vi "camara.vi"() -> ()   [LabVIEW 2010]
uses:
  <vilib>/addons/PixeLINK/Low Level Functions/ACQUISITION.llb/TDPU-Acquisition-StreamState.ctl
  <vilib>/addons/PixeLINK/Low Level Functions/CAMERA_FEATURES.llb/TDPU-CameraFeatures-FeatureIds.ctl
panel:
  out "output array":u8[][](array[numeric])
  out "unsigned 32bit integer":u32
  out "ROI y":dbl
  out "ROI x":dbl
  in  "Error IN":errorcluster
  out "Error OUT":errorcluster
  in  "error in (no error)":errorcluster
  out "error out":errorcluster
  out "Image":T1(plugin-control)
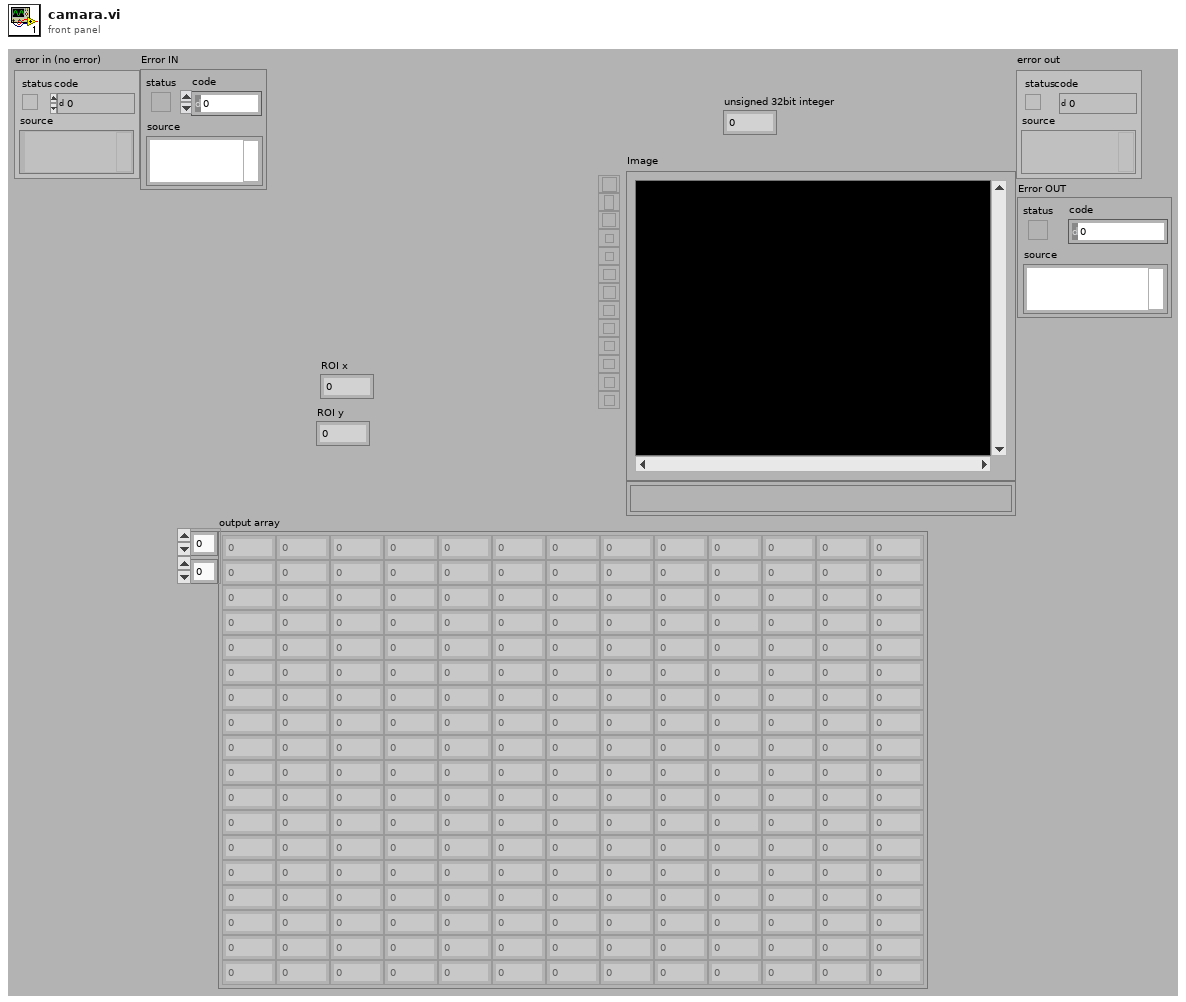
[diagram p1: front panel]
types:
  T1 = typedef "IMAQ Image.ctl" = refnum<image>
  T2 = typedef "TDPU-Acquisition-StreamState.ctl" = u32
  T3 = typedef "TDPU-CameraFeatures-FeatureIds.ctl" = u32
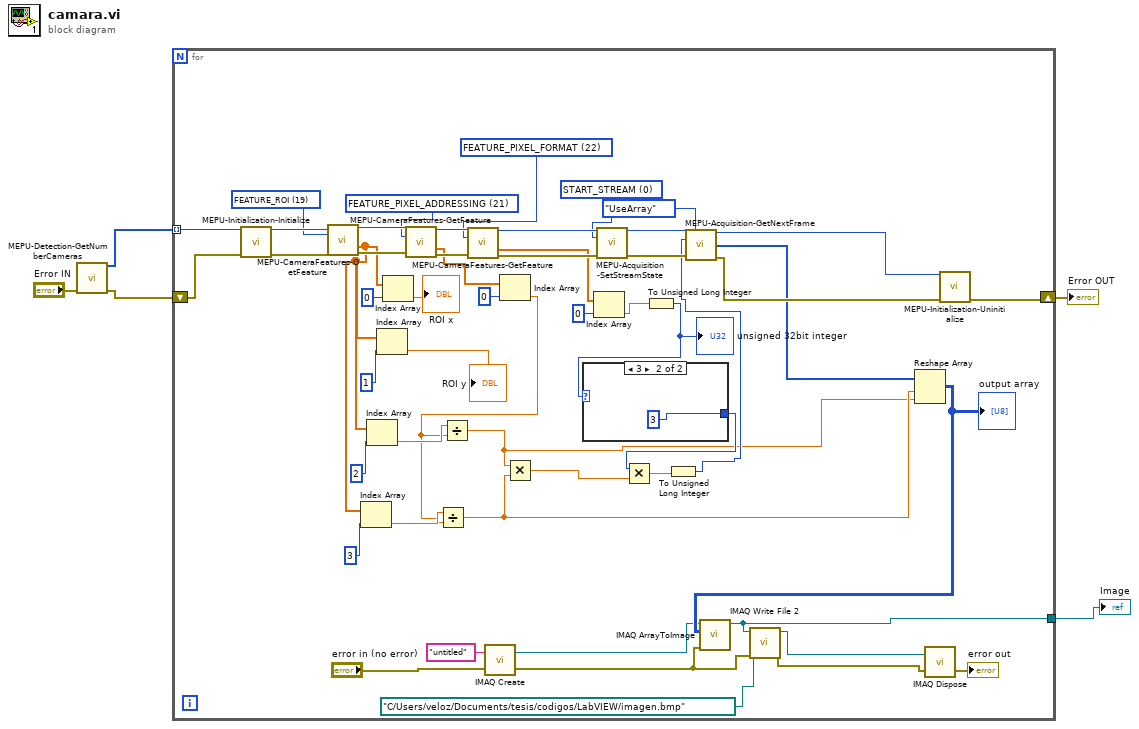
[diagram p0: block diagram]
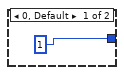
[diagram p2: hidden frame]
diagram:
  n1 = call <vilib>:"MEPU-Detection-GetNumberCameras.vi"("Error IN"="Error IN") -> ("LV_SerialNumbers OUT"=w2:u32[], "Error OUT"=w5:errorcluster)  [unwired: 12 in, 1 out]
  n2 = for {
    shift-right: [w54] -> w4
    shift-left: w5 -> [w55]
    tunnel: w2 -> [w53] mode=indexing
    tunnel: [w12] -> w1
    w18 = T2 0 items=["START_STREAM", "PAUSE_STREAM", "STOP_STREAM"] ("uStreamState IN")
    w22 = T3 22 items=["FEATURE_BRIGHTNESS", "FEATURE_EXPOSURE", "FEATURE_SHARPNESS", "FEATURE_WHITE_BAL", "FEATURE_HUE", "FEATURE_SATURATION", "FEATURE_GAMMA", "FEATURE_SHUTTER", "FEATURE_GAIN", "FEATURE_IRIS", "FEATURE_FOCUS", "FEATURE_TEMPERATURE", "FEATURE_TRIGGER", "FEATURE_ZOOM", "FEATURE_PAN", "FEATURE_TILT", "FEATURE_OPT_FILTER", "FEATURE_GPIO", "FEATURE_FRAME_RATE", "FEATURE_ROI", "FEATURE_FLIP", "FEATURE_PIXEL_ADDRESSING", "FEATURE_PIXEL_FORMAT", "FEATURE_EXTENDED_SHUTTER", "FEATURE_AUTO_ROI", "FEATURE_LOOKUP_TABLE", "FEATURE_MEMORY_CHANNEL", "FEATURE_WHITE_SHADING", "FEATURE_ROTATE", "FEATURE_IMAGER_CLK_DIVISOR", "FEATURE_TRIG_WITH_CNTRLD_LIGHT", "FEATURE_MAX_PIXEL_SIZE"] ("uFeatureId IN")
    w32 = T3 21 items=["FEATURE_BRIGHTNESS", "FEATURE_EXPOSURE", "FEATURE_SHARPNESS", "FEATURE_WHITE_BAL", "FEATURE_HUE", "FEATURE_SATURATION", "FEATURE_GAMMA", "FEATURE_SHUTTER", "FEATURE_GAIN", "FEATURE_IRIS", "FEATURE_FOCUS", "FEATURE_TEMPERATURE", "FEATURE_TRIGGER", "FEATURE_ZOOM", "FEATURE_PAN", "FEATURE_TILT", "FEATURE_OPT_FILTER", "FEATURE_GPIO", "FEATURE_FRAME_RATE", "FEATURE_ROI", "FEATURE_FLIP", "FEATURE_PIXEL_ADDRESSING", "FEATURE_PIXEL_FORMAT", "FEATURE_EXTENDED_SHUTTER", "FEATURE_AUTO_ROI", "FEATURE_LOOKUP_TABLE", "FEATURE_MEMORY_CHANNEL", "FEATURE_WHITE_SHADING", "FEATURE_ROTATE", "FEATURE_IMAGER_CLK_DIVISOR", "FEATURE_TRIG_WITH_CNTRLD_LIGHT", "FEATURE_MAX_PIXEL_SIZE"] ("uFeatureId IN")
    w40 = T3 19 items=["FEATURE_BRIGHTNESS", "FEATURE_EXPOSURE", "FEATURE_SHARPNESS", "FEATURE_WHITE_BAL", "FEATURE_HUE", "FEATURE_SATURATION", "FEATURE_GAMMA", "FEATURE_SHUTTER", "FEATURE_GAIN", "FEATURE_IRIS", "FEATURE_FOCUS", "FEATURE_TEMPERATURE", "FEATURE_TRIGGER", "FEATURE_ZOOM", "FEATURE_PAN", "FEATURE_TILT", "FEATURE_OPT_FILTER", "FEATURE_GPIO", "FEATURE_FRAME_RATE", "FEATURE_ROI", "FEATURE_FLIP", "FEATURE_PIXEL_ADDRESSING", "FEATURE_PIXEL_FORMAT", "FEATURE_EXTENDED_SHUTTER", "FEATURE_AUTO_ROI", "FEATURE_LOOKUP_TABLE", "FEATURE_MEMORY_CHANNEL", "FEATURE_WHITE_SHADING", "FEATURE_ROTATE", "FEATURE_IMAGER_CLK_DIVISOR", "FEATURE_TRIG_WITH_CNTRLD_LIGHT", "FEATURE_MAX_PIXEL_SIZE"] ("uFeatureId IN")
    n3 = call <vilib>:"MEPU-Initialization-Initialize.vi"("uSerialNumber IN"=w53, "Error IN"=w55) -> ("phCamera OUT"=w52:u32, "Error OUT"=w49:errorcluster)  [unwired: 11 in, 1 out]
    n4 = call <vilib>:"MEPU-CameraFeatures-GetFeature.vi"("hCamera IN"=w52, "uFeatureId IN"=w40, "Error IN"=w49) -> ("hCamera OUT"=w51:u32, "pParms OUT"=w33:dbl[], "Error OUT"=w48:errorcluster)  [unwired: 8 in, 2 out]
    n5 = Index Array(array=w33, index=3) -> (element=w28:dbl)
    n6 = Index Array(array=w33, index=2) -> (element=w29:dbl)
    n7 = Index Array(array=w33, index=1) -> (element=→"ROI y":dbl)
    n8 = Index Array(array=w33, index=0) -> (element=→"ROI x":dbl)
    n9 = call <vilib>:"MEPU-CameraFeatures-GetFeature.vi"("hCamera IN"=w51, "uFeatureId IN"=w32, "Error IN"=w48) -> ("hCamera OUT"=w50:u32, "pParms OUT"=w31:dbl[], "Error OUT"=w47:errorcluster)  [unwired: 8 in, 2 out]
    n10 = call <vilib>:"MEPU-CameraFeatures-GetFeature.vi"("hCamera IN"=w50, "uFeatureId IN"=w22, "Error IN"=w47) -> ("hCamera OUT"=w43:u32, "pParms OUT"=w25:dbl[], "Error OUT"=w46:errorcluster)  [unwired: 8 in, 2 out]
    n11 = call "IMAQ Create"("Image Name"="untitled", "error in (no error)"="error in (no error)") -> ("New Image"=w13:T1, "error out"=w9:errorcluster)  [unwired: 3 in]
    n12 = Index Array(array=w31, index=0) -> (element=w27:dbl)
    n13 = Divide(x=w28, y=w27) -> (x/y=w7:dbl)
    n14 = Divide(x=w29, y=w27) -> (x/y=w6:dbl)
    n15 = Multiply(x=w6, y=w7) -> (x*y=w21:dbl)
    n16 = Index Array(array=w25, index=0) -> (element=w24:dbl)
    n17 = call <vilib>:"MEPU-Acquisition-SetStreamState.vi"("hCamera IN"=w43, "uStreamState IN"=w18, "Error IN"=w46) -> ("hCamera OUT"=w42:u32, "Error OUT"=w45:errorcluster)  [unwired: 11 in]
    n18 = To Unsigned Long Integer(number=w24) -> (unsigned 32bit integer=w23:u32)
    "unsigned 32bit integer" <- w23
    n19 = case shown="3" w23 {
      tunnel: [1 3] -> w20
      frame 0, Default {
      }
      frame 3 {
      }
    }
    n20 = Multiply(x=w20, y=w21) -> (x*y=w19:dbl)
    n21 = To Unsigned Long Integer(number=w19) -> (unsigned 32bit integer=w16:u32)
    n22 = call <vilib>:"MEPU-Acquisition-GetNextFrame.vi"("hCamera IN"=w42, "Mode IN"=enum16{"UseArray", "UsePointer"}."UseArray", "uBufferSize IN"=w16, "Error IN"=w45) -> ("hCamera OUT"=w41:u32, "Data OUT"=w14:u8[], "Error OUT"=w44:errorcluster)  [unwired: 7 in, 2 out]
    n23 = Reshape Array(w14, w7, w6) -> (w15:u8[][])
    "output array" <- w15
    n24 = call "IMAQ ArrayToImage"("error in (no error)"=w9, "Image Pixels (U8)"=w15, "Image"=w13) -> ("Image Out"=w12:T1)  [unwired: 7 in, 1 out]
    n25 = call-poly "IMAQ Write File 2"("error in (no error)"=w9, "File Path"=path "C:/Users/veloz/Documents/tesis/codigos/LabVIEW/imagen.bmp", "Image"=w12) -> ("error out"=w10:errorcluster, "Image Out (duplicate)"=w11:T1)  [unwired: 7 in]
    n26 = call "IMAQ Dispose"("Image"=w11, "error in (no error)"=w10) -> ("error out"=→"error out":errorcluster)  [unwired: 4 in]
    n27 = call <vilib>:"MEPU-Initialization-Uninitialize.vi"("hCamera IN"=w41, "Error IN"=w44) -> ("Error OUT"=w54:errorcluster)  [unwired: 13 in]
  }
  "Error OUT" <- w4
  "Image" <- w1
